vi "Set Motors.vi"(8 "error in (no error)":errorcluster, 10 "motors":refnum<class "NI_Robotics_KUKA youBot Arm Motor.lvclass">[](array[class]), 11 "KUKA youBot arm in":refnum<class "NI_Robotics_KUKA youBot Arm.lvclass">) -> (0 "error out":errorcluster, 3 "KUKA youBot arm out":refnum<class "NI_Robotics_KUKA youBot Arm.lvclass">)   [LabVIEW 2017, in "NI_Robotics_KUKA youBot Host.lvlib" / "NI_Robotics_KUKA youBot Arm.lvclass"]
uses:
  <vilib>/robotics/KUKA youBot/Basic Device/Arm/NI_Robotics_KUKA youBot Arm.lvclass
  <vilib>/robotics/KUKA youBot/Motor/Arm Motor/NI_Robotics_KUKA youBot Arm Motor.lvclass
  <vilib>/robotics/KUKA youBot/Basic Device/Arm/NI_Robotics_KUKA youBot Arm.lvclass/NI_Robotics_KUKA youBot Arm.ctl
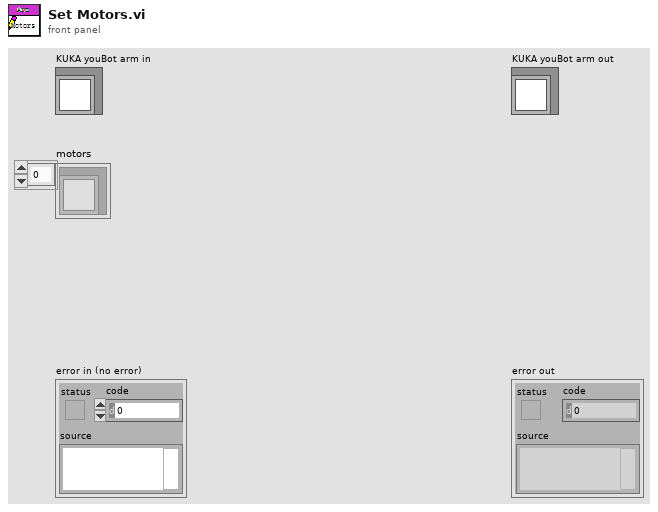
[diagram p1: front panel]
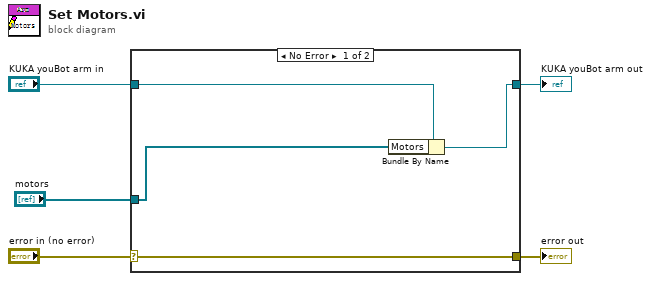
[diagram p0: block diagram]
diagram:
  n1 = case shown="No Error" "error in (no error)" {
    selector: "error in (no error)" -> [w9 w10]
    tunnel: [w9 w10] -> w4
    tunnel: [w8 w11] -> w2
    tunnel: "KUKA youBot arm in" -> [w7 w11]
    tunnel: "motors" -> [w6 _]
    frame No Error {
      n2 = Bundle By Name(cluster=w7, "Motors"=w6) -> (w8:refnum<class "NI_Robotics_KUKA youBot Arm.lvclass">)
    }
    frame Error {
    }
  }
  "error out" <- w4
  "KUKA youBot arm out" <- w2
